vi "index to target.vi"(11 "i32":i32) -> (3 "target":T1)   [LabVIEW 2013, in "TBM configuration.lvclass"]
doc: "Converts an index (I32) to a target (U16) for safe use in for loops and other indexing scenarios."
uses:
  TBM configuration.lvclass
  Target Types.ctl
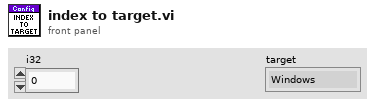
[diagram p1: front panel]
types:
  T1 = typedef "TBM configuration.lvclass/Target Types.ctl" = enum16{"Windows", "Mac", "Linux", "Linux RT ARM", "VxWorks", "Pharlap", "Other", "Linux RT x64"}
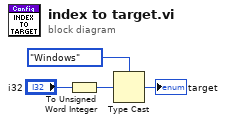
[diagram p0: block diagram]
diagram:
  n1 = To Unsigned Word Integer(number="i32") -> (unsigned 16bit integer=w1:u16)
  n2 = Type Cast(type=Target_Types."Windows" ("Target Types"), x=w1) -> (*(type *) &x=→"target":T1)
